vi "MFP assistant - Lead number to channel converter.vi"(11 "Lead number":dbl) -> (3 "Channel number (0, 1, 2,...)":dbl)   [LabVIEW 2016]
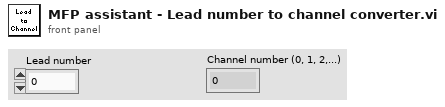
[diagram p1: front panel]
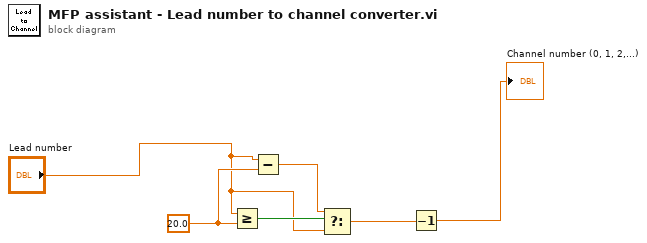
[diagram p0: block diagram]
diagram:
  w5 = 20.0 ("y")
  n1 = Greater Or Equal?(x="Lead number", y=w5) -> (x >= y?=w6:bool)
  n2 = Subtract(x="Lead number", y=w5) -> (x-y=w2:dbl)
  n3 = Select(t=w2, s=w6, f="Lead number") -> (s? t:f=w3:dbl)
  n4 = Decrement(x=w3) -> (x-1=→"Channel number (0, 1, 2,...)":dbl)
